vi "LabVIEW SubVI autogen Name Prefix.vi"() -> (0 "datatype prefix":string="LVSubVI_")   [LabVIEW 2018]
doc: "Returns prefix for autogeneratted names for SubVI."
panel:
  # "Prefix stored in this VI as default value."
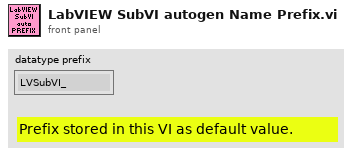
[diagram p1: front panel]
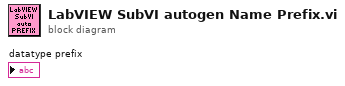
[diagram p0: block diagram]
diagram:
